vi "Write Matching Devices.vi"(10 "Matching Devices":string[](array[string]), 11 "Respond with Devices for Measurement Msg in":refnum<class "Respond with Devices for Measurement Msg.lvclass">) -> (3 "Respond with Devices for Measurement Msg out":refnum<class "Respond with Devices for Measurement Msg.lvclass">)   [LabVIEW 2015, in "Controller Actor.lvlib" / "Respond with Devices for Measurement Msg.lvclass"]
uses:
  Respond with Devices for Measurement Msg.lvclass
  Respond with Devices for Measurement Msg.lvclass/Respond with Devices for Measurement Msg.ctl
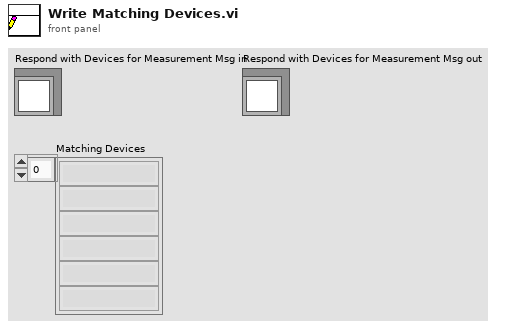
[diagram p1: front panel]
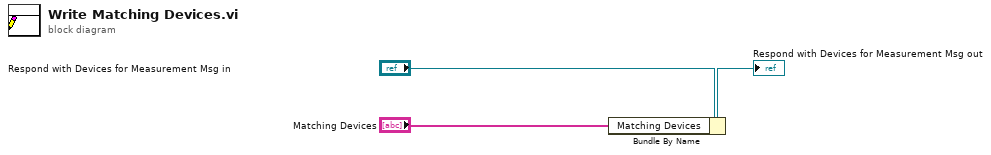
[diagram p0: block diagram]
diagram:
  n1 = Bundle By Name(cluster="Respond with Devices for Measurement Msg in", "Matching Devices"="Matching Devices") -> (→"Respond with Devices for Measurement Msg out":refnum<class "Respond with Devices for Measurement Msg.lvclass">)
